vi "Shoulder Call.vi"(3 "Joystick Axes":dbl[](array[numeric])) -> ()   [LabVIEW 2018]
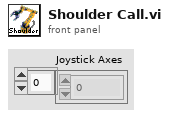
[diagram p1: front panel]
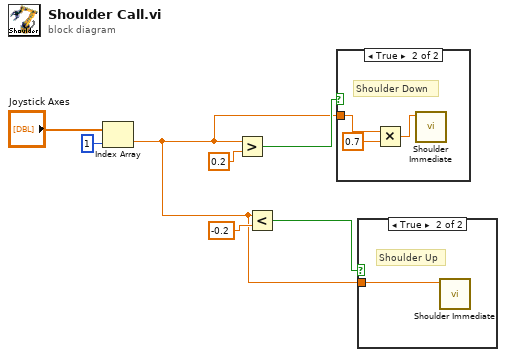
[diagram p0: block diagram]
diagram:
  n1 = Index Array(array="Joystick Axes", index=1) -> (element=w1:dbl)
  n2 = Greater?(x=w1, y=0.2) -> (0:w2:bool)
  n3 = Less?(x=w1, y=-0.2) -> (x < y?=w3:bool)
  n4 = case shown="True" w2 {
    tunnel: w1 -> [_ w10]
    frame False {
    }
    frame True {
      # "Shoulder Down"
      n5 = Multiply(x=w10, y=0.7) -> (x*y=w8:dbl)
      n6 = call "Shoulder Immediate.vi"("Setpoint"=w8) -> ()  [unwired: 10 in, 1 out]
    }
  }
  n7 = case shown="True" w3 {
    tunnel: w1 -> [_ w11]
    frame False {
    }
    frame True {
      # "Shoulder Up"
      n8 = call "Shoulder Immediate.vi"("Setpoint"=w11) -> ()  [unwired: 10 in, 1 out]
    }
  }
